vi "PaintFindedDisplac1.vi"(2 "error IN":errorcluster, 3 "Array of Points IN":dbl[](array[numeric]), 4 "Image IN":T1) -> (0 "error OUT":errorcluster, 1 "Image OUT":T1)   [LabVIEW 2017]
uses:
  <vilib>/vision/Image Controls.llb/IMAQ Image.ctl
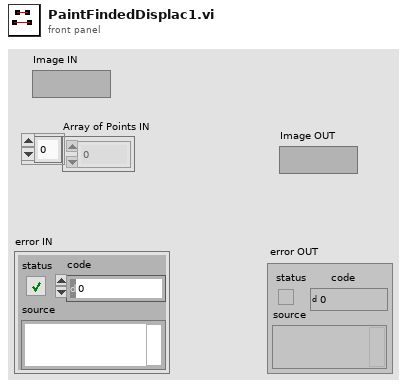
[diagram p1: front panel]
types:
  T1 = typedef "IMAQ Image.ctl" = refnum<image>
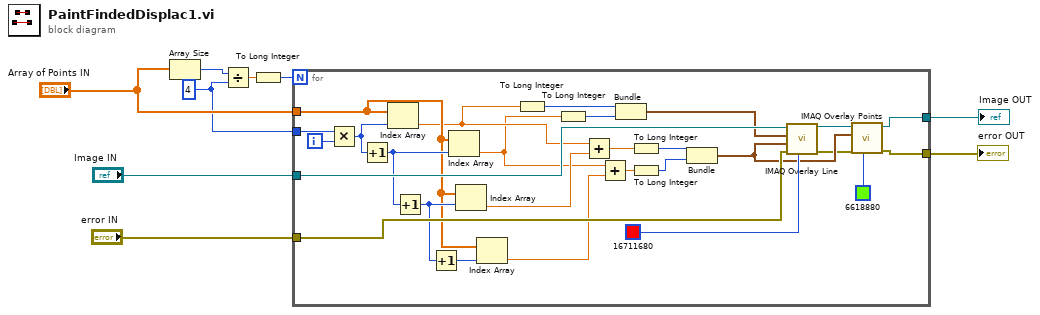
[diagram p0: block diagram]
diagram:
  w3 = 4 ("y")
  n1 = Array Size(array="Array of Points IN") -> (size(s)=w9:i32)
  n2 = Divide(x=w9, y=w3) -> (x/y=w2:dbl)
  n3 = To Long Integer(number=w2) -> (32bit integer=w1:i32)
  n4 = for {
    N: w1 -> [_]
    tunnel: "Image IN" -> [w34]
    tunnel: "Array of Points IN" -> [w31]
    tunnel: "error IN" -> [w35]
    tunnel: [w24] -> w5
    tunnel: [w22] -> w4
    tunnel: w3 -> [w17]
    i -> [w18]
    n5 = Multiply(x=w17, y=w18) -> (x*y=w15:i32)
    n6 = Increment(x=w15) -> (x+1=w33:i32)
    n7 = Index Array(array=w31, index=w15) -> (element=w13:dbl)
    n8 = Increment(x=w33) -> (x+1=w32:i32)
    n9 = Increment(x=w32) -> (x+1=w14:i32)
    n10 = Index Array(array=w31, index=w33) -> (element=w11:dbl)
    n11 = Index Array(array=w31, index=w32) -> (element=w29:dbl)
    n12 = Index Array(array=w31, index=w14) -> (element=w28:dbl)
    n13 = To Long Integer(number=w13) -> (32bit integer=w12:i32)
    n14 = To Long Integer(number=w11) -> (32bit integer=w10:i32)
    n15 = Add(x=w13, y=w29) -> (x+y=w19:dbl)
    n16 = Add(x=w11, y=w28) -> (x+y=w21:dbl)
    n17 = Bundle(w12, w10) -> (w30:cluster{i32, i32})  [unwired: 1 in]
    n18 = To Long Integer(number=w19) -> (32bit integer=w16:i32)
    n19 = To Long Integer(number=w21) -> (32bit integer=w20:i32)
    n20 = Bundle(w16, w20) -> (w26:cluster{i32, i32})  [unwired: 1 in]
    n21 = call "IMAQ Overlay Line"("Color"=u32 16711680, "error in (no error)"=w35, "End Point"=w26, "Start Point"=w30, "Image"=w34) -> ("error out"=w23:errorcluster, "Image Out"=w27:T1)  [unwired: 5 in]
    n22 = call "IMAQ Overlay Points"("Color"=u32 6618880, "error in (no error)"=w23, "Point"=w26, "Image"=w27) -> ("error out"=w22:errorcluster, "Image Out"=w24:T1)  [unwired: 6 in]
  }
  "Image OUT" <- w5
  "error OUT" <- w4
